vi "Weibull CDF.vi"(9 "b":dbl=3.0, 10 "a":dbl=1.0, 11 "x":dbl=1.0) -> (0 "error":i32, 3 "cdf(x)":dbl=0.6321205588285577)   [LabVIEW 2017, in "NI_Gmath.lvlib"]
doc: "Computes the continuous cumulative distribution function (CDF), or the probability that the random variate X, where X describes the selected distribution type, has a value less than or equal to <B>x</B>. You must manually select the polymorphic instance to use."
uses:
  <vilib>/gmath/NI_Gmath.lvlib
  <vilib>/gmath/statdist.llb/st_error_code.ctl
panel:
  # "Weibull CDF"
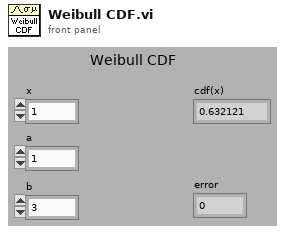
[diagram p1: front panel]
types:
  T1 = typedef "NI_Gmath.lvlib/st_error_code.ctl" = i32
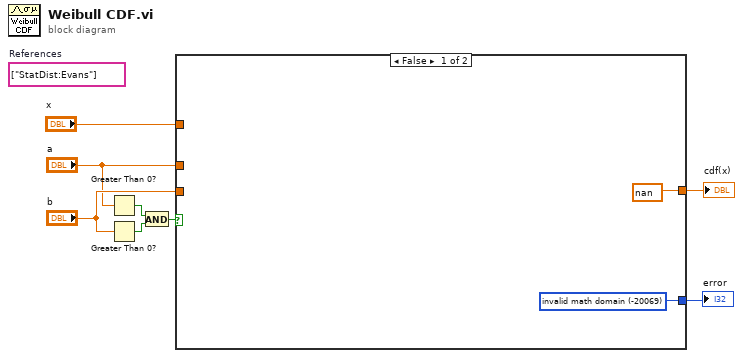
[diagram p0: block diagram]
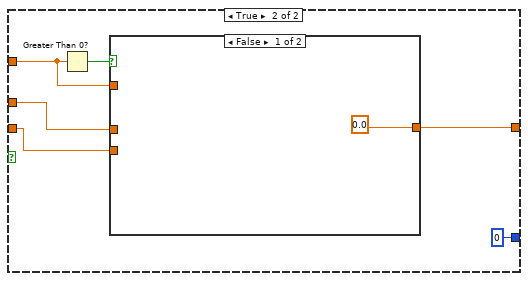
[diagram p2: hidden frame]
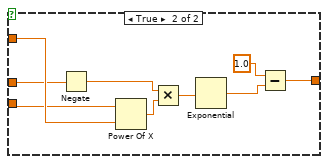
[diagram p3: hidden frame]
diagram:
  (unwired) string[] ["StatDist:Evans"]  # References
  n1 = Greater Than 0?(x="a") -> (x > 0?=w3:bool)
  n2 = Greater Than 0?(x="b") -> (x > 0?=w4:bool)
  n3 = And(x=w3, y=w4) -> (x .and. y?=w5:bool)
  n4 = case shown="False" w5 {
    tunnel: "b" -> [_ w11]
    tunnel: [w9 0 ("invalid math domain")] -> w8
    tunnel: [nan w14] -> w7
    tunnel: "x" -> [_ w13]
    tunnel: "a" -> [_ w12]
    frame False {
      w9 = T1 -20069 items=["invalid math domain"=-20069, "Fourier interpolation size m >= n"=-20070, "empty array"=-20003] ("stat interp error code")
    }
    frame True {
      n5 = Greater Than 0?(x=w13) -> (x > 0?=w15:bool)
      n6 = case shown="False" w15 {
        tunnel: [0.0 w18] -> w14
        tunnel: w13 -> [_ w25]
        tunnel: w12 -> [_ w23]
        tunnel: w11 -> [_ w24]
        frame False {
        }
        frame True {
          n7 = Negate(x=w23) -> (-x=w21:dbl)
          n8 = Power Of X(1:w25, 2:w24) -> (0:w22:dbl)
          n9 = Multiply(x=w21, y=w22) -> (x*y=w20:dbl)
          n10 = Exponential(1:w20) -> (0:w19:dbl)
          n11 = Subtract(x=1.0, y=w19) -> (x-y=w18:dbl)
        }
      }
    }
  }
  "cdf(x)" <- w7
  "error" <- w8
